vi "Riccati_DARE_Iterate.vi"(8 "R":T1, 9 "Q":T1, 10 "B":T1, 11 "A":T1) -> (0 "error out":errorcluster, 1 "Error":bool, 2 "Iterations":i32, 3 "Answer":T1)   [LabVIEW 2019, in "Trajectory_Library.lvlib"]
doc: "Solves the discrete alegebraic Riccati equation.\n\nThis uses an iterative method to arrive at the solution. Run time is not deterministic and this routine should not be used during run-time, only during initialization.\n \nInput:\n - A -- System matrix.\n - B -- nput matrix.\n - Q -- State cost matrix.\n - R -- Input cost matrix.\n\nOutputs:\n Answer -- Solution of DARE.\n iterations -- Number of iterations\n error -- If TRUE, an error occured"
uses:
  Trajectory_Library.lvlib
  <vilib>/Analysis/Matrix/Datatypes/RealMatrix.ctl
  <vilib>/Analysis/7linalg.llb/Real Transpose Matrix.vi
  <vilib>/Analysis/baseanly.llb/Real A x B.vi
  <vilib>/Analysis/baseanly.llb/Real Inverse Matrix.vi
  <vilib>/Analysis/Matrix/Numeric/Add/Add - RM,RM.vi
  <vilib>/Analysis/Matrix/Numeric/Subtract/Subtract - RM,RM.vi
  <vilib>/Analysis/Matrix/Numeric/Multiply/Multiply - RM,R.vi
  <vilib>/Analysis/NI_AALPro.lvlib
  <vilib>/Analysis/NI_AALBase.lvlib
  <vilib>/Analysis/Matrix/NI_Matrix.lvlib
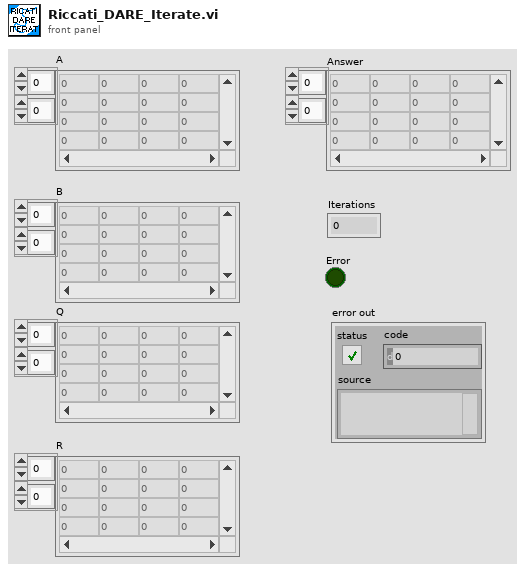
[diagram p1: front panel]
types:
  T1 = typedef "NI_Matrix.lvlib/RealMatrix.ctl" = dbl[][]
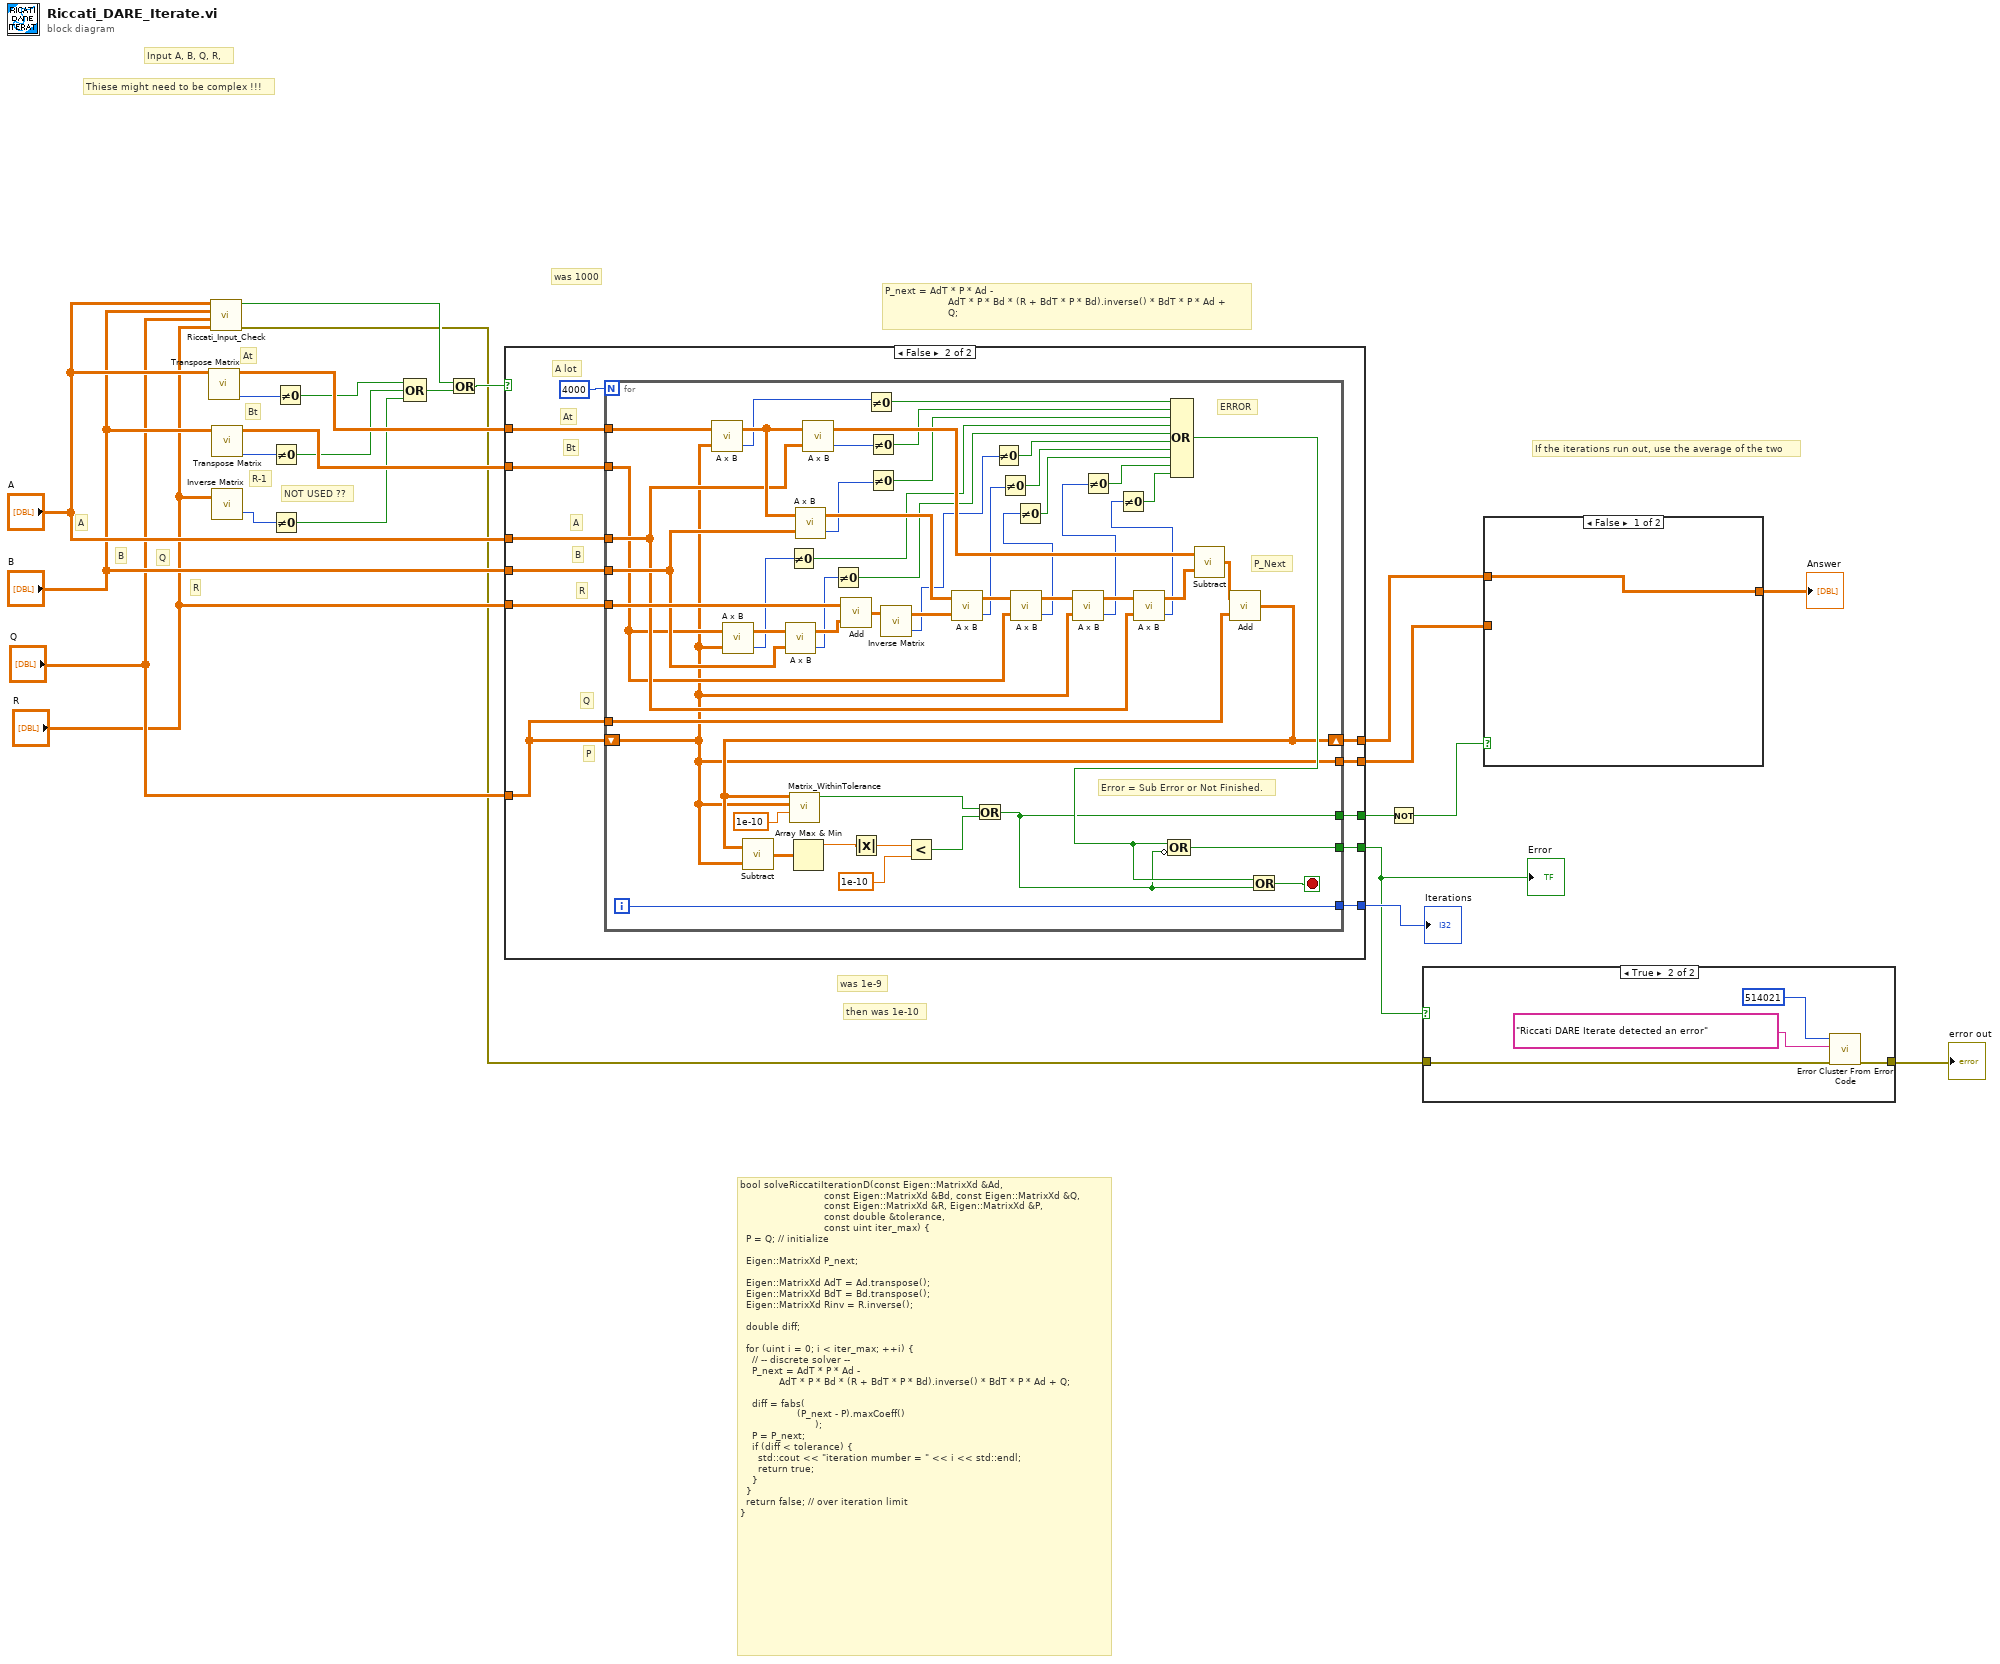
[diagram p0: block diagram]
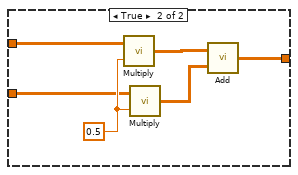
[diagram p2: hidden frame]
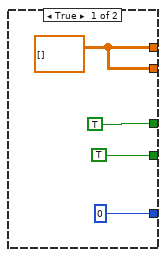
[diagram p4: hidden frame]
diagram:
  # "If the iterations run out, use the average of the two"
  # "then was 1e-10"
  # "was 1000"
  # "was 1e-9"
  # "NOT USED ??"
  # "P_next = AdT * P * Ad -\n                     AdT * P * Bd * (R + BdT * P * Bd).inverse() * BdT * P * Ad + \n                     Q;"
  # "B"
  # "R-1"
  # "Bt"
  # "At"
  # "bool solveRiccatiIterationD(const Eigen::MatrixXd &Ad,\n                            const Eigen::MatrixXd &Bd, const Eigen::MatrixXd &Q,\n                            const Eigen::MatrixXd &R, Eigen::MatrixXd &P,\n                            const double &tolerance,\n                            const uint iter_max) {\n  P = Q; // initialize\n\n  Eigen::MatrixXd P_next;\n\n  Eigen::MatrixXd AdT = Ad.transpose();\n  Eigen::MatrixXd BdT = Bd.transpose();\n  Eigen::MatrixXd Rinv = R.inverse();\n\n  double diff;\n\n  for (uint i = 0; i < iter_max; ++i) {\n    // -- discrete solver --\n    P_next = AdT * P * Ad -\n             AdT * P * Bd * (R + BdT * P * Bd).inverse() * BdT * P * Ad + Q;\n\n    diff = fabs(    \n                   (P_next - P).maxCoeff()\n                         );\n    P = P_next;\n    if (diff < tolerance) {\n      std::cout << \"iteration mumber = \" << i << std::endl;\n      return true;\n    }\n  }\n  return false; // over iteration limit\n}"
  # "R"
  # "Q"
  # "A"
  # "Thiese might need to be complex !!!"
  # "Input A, B, Q, R,"
  n1 = call-poly <vilib>:"Transpose Matrix.vi"("Input Matrix"="A") -> ("error"=w20:i32, "Matrix Transpose"=w24:T1)  [unwired: 9 in]
  n2 = call "Riccati_Input_Check.vi"("R"="R", "Q"="Q", "B"="B", "A"="A") -> ("error out"=w7:errorcluster, "Error"=w10:bool)  [unwired: 6 in]
  n3 = call-poly <vilib>:"Transpose Matrix.vi"("Input Matrix"="B") -> ("error"=w19:i32, "Matrix Transpose"=w23:T1)  [unwired: 9 in]
  n4 = call-poly <vilib>:"Inverse Matrix.vi"("Input Matrix"="R") -> ("error"=w21:i32)  [unwired: 1 in, 1 out]
  n5 = Not Equal To 0?(x=w19) -> (x != 0?=w17:bool)
  n6 = Not Equal To 0?(x=w21) -> (x != 0?=w18:bool)
  n7 = Not Equal To 0?(x=w20) -> (x != 0?=w16:bool)
  n8 = Compound Arithmetic op=OR(w16, w17, w18) -> (w11:bool)
  n9 = Or(x=w10, y=w11) -> (x .or. y?=w12:bool)
  n10 = case shown="False" w12 {
    tunnel: w24 -> [_ w39]
    tunnel: w23 -> [_ w38]
    tunnel: "R" -> [_ w37]
    tunnel: "A" -> [_ w36]
    tunnel: "B" -> [_ w35]
    tunnel: [w25 w34] -> w3
    tunnel: [0 w33] -> w22
    tunnel: [TRUE w32] -> w8
    tunnel: "Q" -> [_ w31]
    tunnel: [TRUE ("WithinTolerance") w30] -> w5
    tunnel: [w25 w29] -> w1
    frame True {
      w25 = T1 [] ("Q")
    }
    frame False {
      # "Q"
      # "At"
      # "Bt"
      # "R"
      # "B"
      # "A"
      # "P"
      # "A lot"
      n11 = for {
        N: 4000 -> [_]
        shift-right: [w47] -> w34
        shift-left: w31 -> [w44]
        tunnel: w39 -> [w92]
        tunnel: w38 -> [w45]
        tunnel: w37 -> [w90]
        tunnel: w36 -> [w80]
        tunnel: w35 -> [w88]
        tunnel: w31 -> [w79]
        tunnel: [w78] -> w33
        tunnel: [w49] -> w32
        tunnel: [w43] -> w30
        tunnel: [w44] -> w29
        i -> [w78]
        stop <- w70 stop-if-true
        # "Error = Sub Error or Not Finished."
        # "ERROR"
        # "P_Next"
        n12 = call-poly <vilib>:"A x B.vi"("B"=w44, "A"=w92) -> ("error"=w69:i32, "A x B"=w91:T1)
        n13 = call-poly <vilib>:"A x B.vi"("B"=w44, "A"=w45) -> ("error"=w66:i32, "A x B"=w89:T1)
        n14 = call-poly <vilib>:"A x B.vi"("B"=w88, "A"=w89) -> ("error"=w65:i32, "A x B"=w87:T1)
        n15 = Not Equal To 0?(x=w66) -> (x != 0?=w61:bool)
        n16 = call-poly <vilib>:"A x B.vi"("B"=w88, "A"=w91) -> ("error"=w67:i32, "A x B"=w85:T1)
        n17 = call-poly <vilib>:"A x B.vi"("B"=w80, "A"=w91) -> ("error"=w68:i32, "A x B"=w73:T1)
        n18 = Not Equal To 0?(x=w65) -> (x != 0?=w60:bool)
        n19 = call-poly <vilib>:"Add.vi"("Real Matrix B"=w87, "Real Matrix A"=w90) -> ("A + B"=w86:T1)
        n20 = Not Equal To 0?(x=w69) -> (x != 0?=w64:bool)
        n21 = Not Equal To 0?(x=w68) -> (x != 0?=w63:bool)
        n22 = Not Equal To 0?(x=w67) -> (x != 0?=w62:bool)
        n23 = call-poly <vilib>:"Inverse Matrix.vi"("Input Matrix"=w86) -> ("error"=w59:i32, "Inverse Matrix"=w84:T1)  [unwired: 1 in]
        n24 = call-poly <vilib>:"A x B.vi"("B"=w84, "A"=w85) -> ("error"=w57:i32, "A x B"=w83:T1)
        n25 = Not Equal To 0?(x=w59) -> (x != 0?=w58:bool)
        n26 = Not Equal To 0?(x=w57) -> (x != 0?=w55:bool)
        n27 = call-poly <vilib>:"A x B.vi"("B"=w45, "A"=w83) -> ("error"=w56:i32, "A x B"=w82:T1)
        n28 = Not Equal To 0?(x=w56) -> (x != 0?=w54:bool)
        n29 = call-poly <vilib>:"A x B.vi"("B"=w44, "A"=w82) -> ("error"=w53:i32, "A x B"=w81:T1)
        n30 = Not Equal To 0?(x=w53) -> (x != 0?=w51:bool)
        n31 = call-poly <vilib>:"A x B.vi"("B"=w80, "A"=w81) -> ("error"=w52:i32, "A x B"=w72:T1)
        n32 = Not Equal To 0?(x=w52) -> (x != 0?=w50:bool)
        n33 = Compound Arithmetic op=OR(w64, w63, w62, w61, w60, w58, w55, w54, w51, w50) -> (w48:bool)
        n34 = call-poly <vilib>:"Subtract.vi"("Real Matrix B"=w72, "Real Matrix A"=w73) -> ("A - B"=w71:T1)
        n35 = call-poly <vilib>:"Add.vi"("Real Matrix B"=w79, "Real Matrix A"=w71) -> ("A + B"=w47:T1)
        n36 = call-poly <vilib>:"Subtract.vi"("Real Matrix B"=w44, "Real Matrix A"=w47) -> ("A - B"=w77:T1)
        n37 = call "Matrix_WithinTolerance.vi"("Tolerance"=1e-10, "Matrix B"=w44, "Matrix A"=w47) -> ("WithinTolerance"=w41:bool)  [unwired: 7 in, 1 out]
        n38 = Array Max & Min(array=w77) -> (max value=w76:dbl)  [unwired: 3 out]
        n39 = Absolute Value(x=w76) -> (abs(x)=w75:dbl)
        n40 = Less?(x=w75, y=1e-10) -> (x < y?=w42:bool)
        n41 = Or(x=w41, y=w42) -> (x .or. y?=w43:bool)
        n42 = Compound Arithmetic op=OR(w48, invert w43) -> (w49:bool)
        n43 = Or(x=w48, y=w43) -> (x .or. y?=w70:bool)
      }
    }
  }
  "Iterations" <- w22
  "Error" <- w8
  n44 = Not(x=w5) -> (.not. x?=w4:bool)
  n45 = case shown="True" w8 {
    tunnel: w7 -> [w93 w94]
    tunnel: [w93 w96] -> w6
    frame False {
    }
    frame True {
      n46 = call <vilib>:"Error Cluster From Error Code.vi"("error in (no error)"=w94, "error message (\"\")"="Riccati DARE Iterate detected an error" ("error message (\"\")"), "error code (0)"=514021) -> ("error out"=w96:errorcluster)  [unwired: 6 in]
    }
  }
  "error out" <- w6
  n47 = case shown="False" w4 {
    tunnel: w3 -> [w98 w103]
    tunnel: [w98 w99] -> w2
    tunnel: w1 -> [_ w102]
    frame False {
    }
    frame True {
      w104 = 0.5
      n48 = call-poly <vilib>:"Multiply.vi"("Real Scalar c"=w104, "Real Matrix A"=w103) -> ("A * c"=w101:T1)
      n49 = call-poly <vilib>:"Multiply.vi"("Real Scalar c"=w104, "Real Matrix A"=w102) -> ("A * c"=w100:T1)
      n50 = call-poly <vilib>:"Add.vi"("Real Matrix B"=w100, "Real Matrix A"=w101) -> ("A + B"=w99:T1)
    }
  }
  "Answer" <- w2
